vi "Lift Controller.vi"(1 "error in":errorcluster, 2 "Button 4":bool, 3 "Button 3":bool) -> (0 "error out":errorcluster)   [LabVIEW 2017]
uses:
  <vilib>/Rock Robotics/WPI/Solenoid/WPI_SolenoidValue.ctl
  <vilib>/Rock Robotics/WPI/Solenoid/WPI_SolenoidGetEnum.vi
  <vilib>/Rock Robotics/WPI/Solenoid/WPI_SolenoidSetEnum.vi
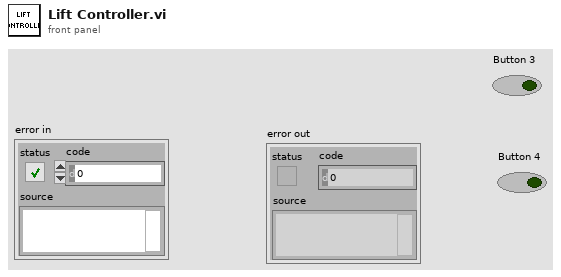
[diagram p1: front panel]
types:
  T1 = typedef "WPI_SolenoidDevRef.ctl" = cluster{"DevStatus":errorcluster, "Pneumatics Control Module":u8, "Forward Solenoid Channel":T2, "Reverse Solenoid Channel":T2}
  T2 = typedef "WPI_SolenoidChannel.ctl" = enum8{"Solenoid 0", "Solenoid 1", "Solenoid 2", "Solenoid 3", "Solenoid 4", "Solenoid 5", "Solenoid 6", "Solenoid 7", "Invalid"}
  T3 = typedef "WPI_SolenoidValue.ctl" = enum16{"Off", "On", "Forward", "Reverse"}
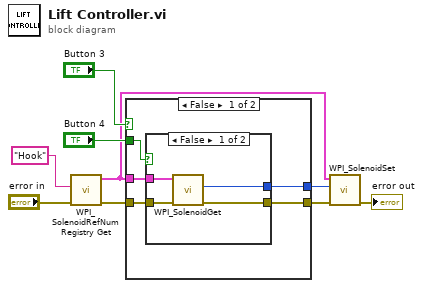
[diagram p0: block diagram]
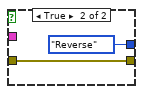
[diagram p2: hidden frame]
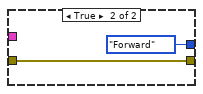
[diagram p3: hidden frame]
diagram:
  n1 = call <vilib>:"WPI_SolenoidRefNum Registry Get.vi"("error in (no error)"="error in", "refnum name"="Hook") -> ("error out"=w2:errorcluster, "SolenoidDevRef"=w4:T1)  [unwired: 8 in]
  n2 = case shown="False" "Button 3" {
    tunnel: [w13 WPI_SolenoidValue."Forward" ("Value")] -> w5
    tunnel: "Button 4" -> [w14 _]
    tunnel: w4 -> [w12 _]
    tunnel: w2 -> [w11 w21]
    tunnel: [w10 w21] -> w1
    frame False {
      n3 = case shown="False" w14 {
        tunnel: [w17 WPI_SolenoidValue."Reverse" ("Value")] -> w13
        tunnel: w12 -> [w18 _]
        tunnel: w11 -> [w16 w19]
        tunnel: [w15 w19] -> w10
        frame False {
          n4 = call-poly <vilib>:"WPI_SolenoidGet.vi"("error in (no error)"=w16, "SolenoidDevRef"=w18) -> ("error out"=w15:errorcluster, "Value"=w17:T3)  [unwired: 7 in, 1 out]
        }
        frame True {
        }
      }
    }
    frame True {
    }
  }
  n5 = call-poly <vilib>:"WPI_SolenoidSet.vi"("error in (no error)"=w1, "Value"=w5, "SolenoidDevRef"=w4) -> ("error out"=→"error out":errorcluster)  [unwired: 7 in, 1 out]
